vi "RobotFPGA.vi"() -> ()   [LabVIEW 2009]
uses:
  <vilib>/eio/EIOMethodNode/EIOMethodNode.xnode
  <vilib>/rvi/eio/nirviEIOMethodImplementation/nirviEIOMethodImplementation.xnode
  <vilib>/rvi/eio/common/nirviEmuTemplateMethod_noerrors.vi
  <vilib>/rvi/eio/common/nirviEmuClasses.ctl
panel:
  in  "PWM9_Enable":bool
  in  "PWM10_Enable":bool
  in  "PWM1_Enable":bool
  in  "PWM2_Enable":bool
  in  "PWM2":cluster{"High (uSec)":u32, "Period (uSec)":u32}
  in  "PWM1":cluster{"High (uSec)":u32, "Period (uSec)":u32}
  in  "PWM10":cluster{"High (uSec)":u32, "Period (uSec)":u32}
  in  "PWM9":cluster{"High (uSec)":u32, "Period (uSec)":u32}
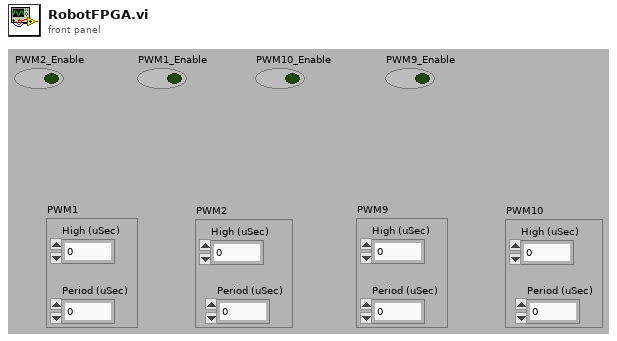
[diagram p1: front panel]
types:
  T1 = typedef "nirviEmuClasses.ctl" = enum16{"IO Read", "IO Write", "Method", "Property Read", "Property Write"}
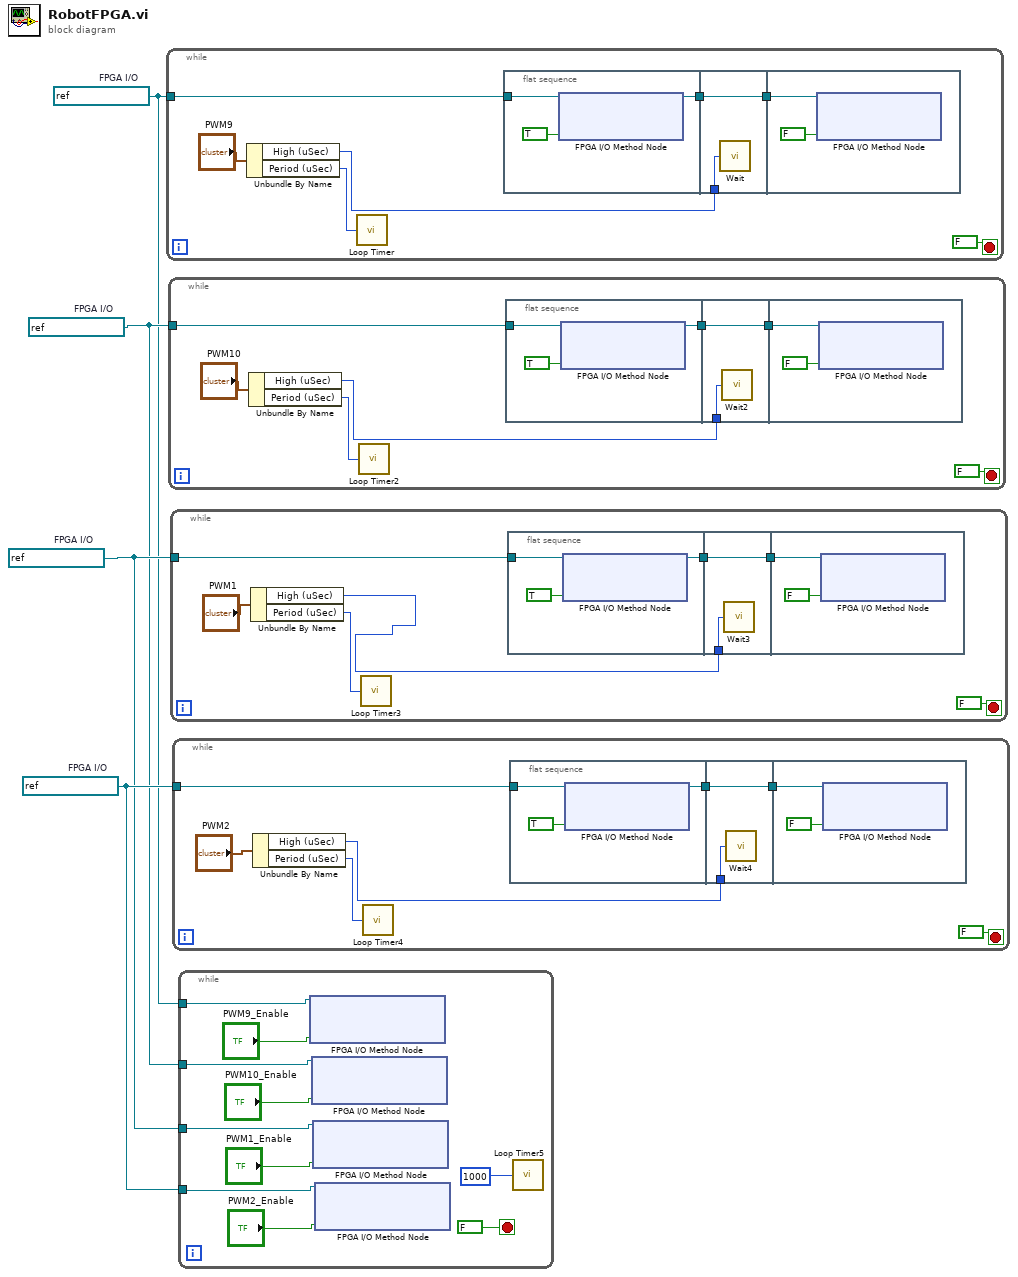
[diagram p0: block diagram]
diagram:
  w4 = refnum<k21> "Mod4/DIO23"  # FPGA I/O
  w3 = refnum<k21> "Mod4/DIO22"  # FPGA I/O
  w2 = refnum<k21> "Mod4/DIO31"  # FPGA I/O
  w1 = refnum<k21> "Mod4/DIO30"  # FPGA I/O
  n1 = while {
    tunnel: w1 -> [w5]
    stop <- FALSE stop-if-true
    n2 = Unbundle By Name("PWM9") -> ("High (uSec)"=w7:u32, "Period (uSec)"=w6:u32)
    n3 = call "Loop Timer"("Count(uSec)"=w6) -> ()  [unwired: 1 out]
    n4 = flat-sequence {
      tunnel: w5 -> [w14]
      tunnel: [w12] -> w10
      tunnel: w10 -> [w27]
      tunnel: [w27] -> w9
      tunnel: w7 -> [w26]
      tunnel: w9 -> [w29]
      frame #0 {
        n5 = xnode "FPGA I/O Method Node"("FPGA I/O In"=w14, "Data"=TRUE) -> ("FPGA I/O Out"=w12:refnum<k21>)
      }
      frame #1 {
        n6 = call "Wait"("Count(uSec)"=w26) -> ()  [unwired: 1 out]
      }
      frame #2 {
        n7 = xnode "FPGA I/O Method Node"("FPGA I/O In"=w29, "Data"=FALSE) -> ()  [unwired: 1 out]
      }
    }
  }
  n8 = while {
    tunnel: w2 -> [w41]
    stop <- FALSE stop-if-true
    n9 = Unbundle By Name("PWM10") -> ("High (uSec)"=w43:u32, "Period (uSec)"=w42:u32)
    n10 = call "Loop Timer2"("Count(uSec)"=w42) -> ()  [unwired: 1 out]
    n11 = flat-sequence {
      tunnel: w41 -> [w50]
      tunnel: [w48] -> w46
      tunnel: w46 -> [w63]
      tunnel: [w63] -> w45
      tunnel: w43 -> [w62]
      tunnel: w45 -> [w65]
      frame #0 {
        n12 = xnode "FPGA I/O Method Node"("FPGA I/O In"=w50, "Data"=TRUE) -> ("FPGA I/O Out"=w48:refnum<k21>)
      }
      frame #1 {
        n13 = call "Wait2"("Count(uSec)"=w62) -> ()  [unwired: 1 out]
      }
      frame #2 {
        n14 = xnode "FPGA I/O Method Node"("FPGA I/O In"=w65, "Data"=FALSE) -> ()  [unwired: 1 out]
      }
    }
  }
  n15 = while {
    tunnel: w3 -> [w79]
    stop <- FALSE stop-if-true
    n16 = Unbundle By Name("PWM1") -> ("High (uSec)"=w78:u32, "Period (uSec)"=w77:u32)
    n17 = call "Loop Timer3"("Count(uSec)"=w77) -> ()  [unwired: 1 out]
    n18 = flat-sequence {
      tunnel: w79 -> [w86]
      tunnel: [w84] -> w82
      tunnel: w82 -> [w99]
      tunnel: [w99] -> w81
      tunnel: w78 -> [w98]
      tunnel: w81 -> [w101]
      frame #0 {
        n19 = xnode "FPGA I/O Method Node"("FPGA I/O In"=w86, "Data"=TRUE) -> ("FPGA I/O Out"=w84:refnum<k21>)
      }
      frame #1 {
        n20 = call "Wait3"("Count(uSec)"=w98) -> ()  [unwired: 1 out]
      }
      frame #2 {
        n21 = xnode "FPGA I/O Method Node"("FPGA I/O In"=w101, "Data"=FALSE) -> ()  [unwired: 1 out]
      }
    }
  }
  n22 = while {
    tunnel: w4 -> [w113]
    stop <- FALSE stop-if-true
    n23 = Unbundle By Name("PWM2") -> ("High (uSec)"=w115:u32, "Period (uSec)"=w114:u32)
    n24 = call "Loop Timer4"("Count(uSec)"=w114) -> ()  [unwired: 1 out]
    n25 = flat-sequence {
      tunnel: w113 -> [w122]
      tunnel: [w120] -> w118
      tunnel: w118 -> [w135]
      tunnel: [w135] -> w117
      tunnel: w115 -> [w134]
      tunnel: w117 -> [w137]
      frame #0 {
        n26 = xnode "FPGA I/O Method Node"("FPGA I/O In"=w122, "Data"=TRUE) -> ("FPGA I/O Out"=w120:refnum<k21>)
      }
      frame #1 {
        n27 = call "Wait4"("Count(uSec)"=w134) -> ()  [unwired: 1 out]
      }
      frame #2 {
        n28 = xnode "FPGA I/O Method Node"("FPGA I/O In"=w137, "Data"=FALSE) -> ()  [unwired: 1 out]
      }
    }
  }
  n29 = while {
    tunnel: w4 -> [w157]
    tunnel: w3 -> [w152]
    tunnel: w2 -> [w151]
    tunnel: w1 -> [w150]
    stop <- FALSE stop-if-true
    n30 = xnode "FPGA I/O Method Node"("FPGA I/O In"=w150, "Enable"="PWM9_Enable") -> ()  [unwired: 1 out]
    n31 = xnode "FPGA I/O Method Node"("FPGA I/O In"=w151, "Enable"="PWM10_Enable") -> ()  [unwired: 1 out]
    n32 = xnode "FPGA I/O Method Node"("FPGA I/O In"=w152, "Enable"="PWM1_Enable") -> ()  [unwired: 1 out]
    n33 = xnode "FPGA I/O Method Node"("FPGA I/O In"=w157, "Enable"="PWM2_Enable") -> ()  [unwired: 1 out]
    n34 = call "Loop Timer5"("Count(mSec)"=u32 1000) -> ()  [unwired: 1 out]
  }
